vi "Read Deposition notif.vi"(8 "error in (no error)":errorcluster, 11 "BC-Main in":refnum<class "SC-Main.lvclass">) -> (0 "error out":errorcluster, 2 "Deposition notif":refnum<notifier>, 3 "BC-Main out":refnum<class "SC-Main.lvclass">)   [LabVIEW 2013, in "SLMControl.lvlib" / "SC-Main.lvclass"]
uses:
  SC-Main.lvclass
  SC-Main.lvclass/SC-Main.ctl
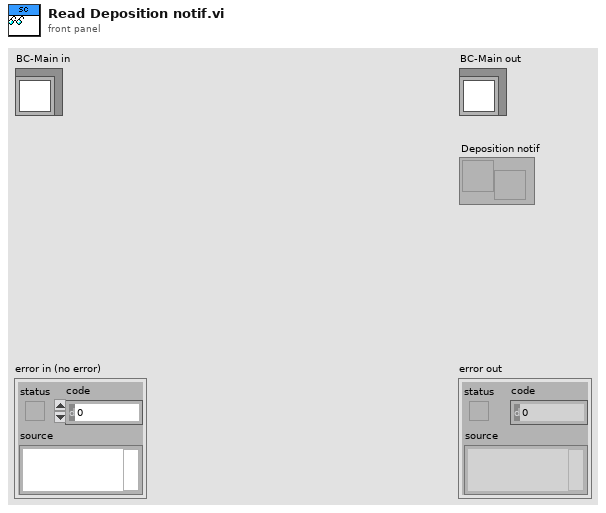
[diagram p1: front panel]
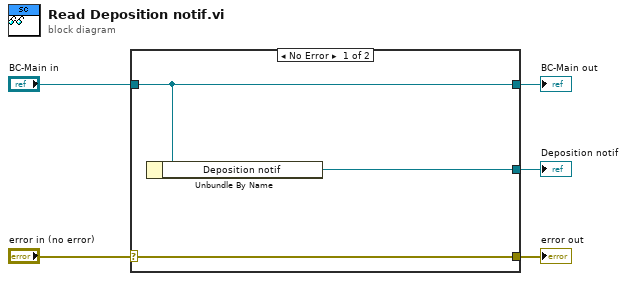
[diagram p0: block diagram]
diagram:
  n1 = case shown="No Error" "error in (no error)" {
    selector: "error in (no error)" -> [w8 w9]
    tunnel: [w8 w9] -> w4
    tunnel: [w7 w10] -> w2
    tunnel: "BC-Main in" -> [w7 w10]
    tunnel: [w6 _] -> w1
    frame No Error {
      n2 = Unbundle By Name(w7) -> ("Deposition notif"=w6:refnum<notifier>)
    }
    frame Error {
    }
  }
  "error out" <- w4
  "BC-Main out" <- w2
  "Deposition notif" <- w1
